vi "anti_wind_up_integral.vi"(7 "Limits":cluster{"Upper limit":dbl, "Lower limit ":dbl}, 8 "Ts":dbl, 9 "Kb":dbl=2000.0 format="%#_13g", 11 "Input":dbl) -> (0 "Integral output":dbl, 3 "Output":dbl)   [LabVIEW 2014]
uses:
  <vilib>/ptbypt/NI_PtbyPt.lvlib
panel:
  # "http://ch.mathworks.com/help/simulink/examples/anti-windup-control-using-a-pid-controller.html"
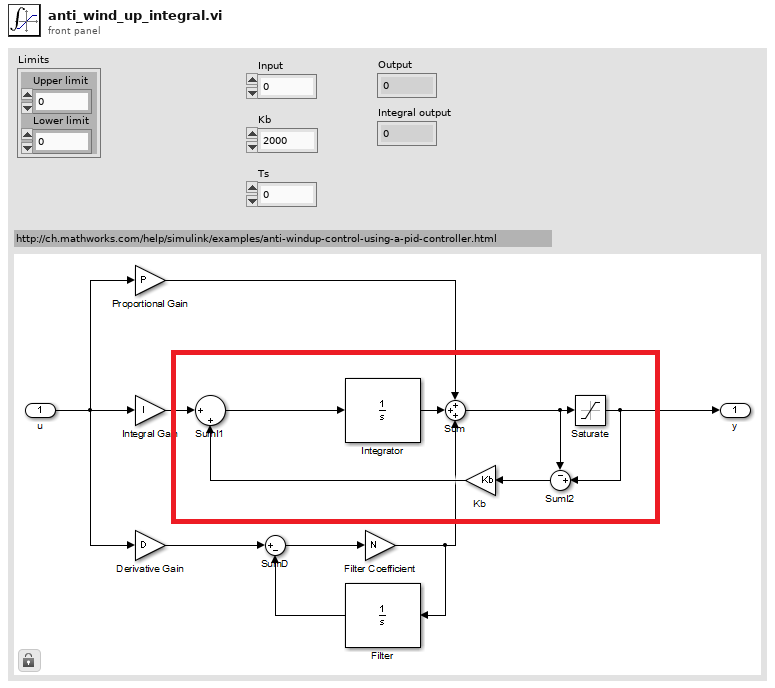
[diagram p1: front panel]
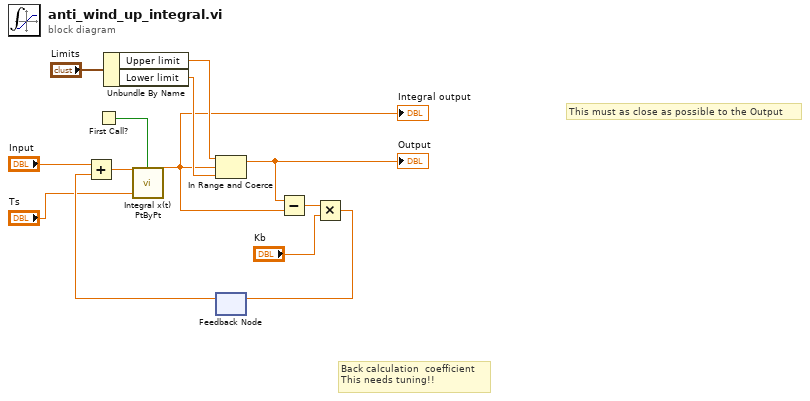
[diagram p0: block diagram]
diagram:
  # "This must as close as possible to the Output"
  # "Back calculation  coefficient\nThis needs tuning!!"
  n1 = First Call?() -> (First Call?: T/F=w8:bool)
  n2 = Unbundle By Name("Limits") -> ("Upper limit"=w2:dbl, "Lower limit"=w3:dbl)
  n3 = feedback #1() -> (w13:dbl)  [unwired: 1 in]
  n4 = Add(x="Input", y=w13) -> (x+y=w11:dbl)
  n5 = call <vilib>:"Integral x(t) PtByPt.vi"("initialize"=w8, "dt"="Ts", "x"=w11) -> ("integral x(t)"=w1:dbl)  [unwired: 1 in, 1 out]
  "Integral output" <- w1
  n6 = In Range and Coerce(upper limit=w2, x=w1, lower limit=w3) -> (coerced(x)=w6:dbl)  [unwired: 1 out]
  "Output" <- w6
  n7 = Subtract(x=w6, y=w1) -> (x-y=w9:dbl)
  n8 = Multiply(x=w9, y="Kb") -> (x*y=w12:dbl)
  n9 = feedback-in #1(w12) -> ()
